vi "Finish.vi"   [LabVIEW 2018]
doc: "This VI is called just before exiting. It is expected to close I/O refnum, save collected data, etc."
uses:
  <vilib>/Rock Robotics/WPI/Utilities/WPI_GetSetVariantRefNum.vi
types:
  T1 = typedef "WPI_CompressorDevRef.ctl" = cluster{"DevStatus":errorcluster, "Pneumatics Control Module":u8}
  T2 = typedef "WPI_RobotDriveDevRef.ctl" = cluster{"DevStatus":errorcluster, "Motors[]":T3[], "Square Inputs":bool, "Max Output":dbl}
  T3 = typedef "WPI_MotorControlDeviceRef.ctl" = cluster{"DeviceStatus":errorcluster, "Type":T4, "PWM":cluster{"PWM Channel":T5, "DeadBand":T6}, "CAN":cluster{"Device Number":u8, "SetOutput VI Ref":variant, "GetOutput VI Ref":variant, "Enable VI Ref":variant, "Disable VI Ref":variant, "Data":variant}, "Invert":bool, "DIO PWM":cluster{"PWM \"Enable\" Channel":T5, "DIOChannel":T7, "PWM Rate":dbl}}
  T4 = typedef "WPI_MotorControlType.ctl" = enum16{"PWM", "CAN", "DIO PWM"}
  T5 = typedef "FPGA_DIOPWMChannel.ctl" = enum8{"PWM 0", "PWM 1", "PWM 2", "PWM 3", "PWM 4", "PWM 5", "PWM 6", "PWM 7", "PWM 8", "PWM 9", "PWM MXP 0", "PWM MXP 1", "PWM MXP 2", "PWM MXP 3", "PWM MXP 4", "PWM MXP 5", "PWM MXP 6", "PWM MXP 7", "PWM MXP 8", "PWM MXP 9", "Invalid"}
  T6 = typedef "WPI_PWMDeadband.ctl" = cluster{"Name":string, "maxPositivePwm":i32, "minPositivePwm":i32, "centerPwm":i32, "maxNegativePwm":i32, "minNegativePwm":i32, "angularRange":u16}
  T7 = typedef "FPGA_DIOChannel.ctl" = enum8{"DIO 0", "DIO 1", "DIO 2", "DIO 3", "DIO 4", "DIO 5", "DIO 6", "DIO 7", "DIO 8", "DIO 9", "DIO MXP 0", "DIO MXP 1", "DIO MXP 2", "DIO MXP 3", "DIO MXP 4", "DIO MXP 5", "DIO MXP 6", "DIO MXP 7", "DIO MXP 8", "DIO MXP 9", "DIO MXP 10", "DIO MXP 11", "DIO MXP 12", "DIO MXP 13", "DIO MXP 14", "DIO MXP 15", "SPI Port CS1", "SPI Port CS2", "SPI Port CS3", "SPI Port MISO", "SPI Port MOSI", "Invalid"}
  T8 = typedef "WPI_EncoderDevRef.ctl" = cluster{"DevStatus":errorcluster, "EncoderIndex":T9, "CounterIndex":T10, "DistancePerCount":dbl, "Decoding Type":T11}
  T9 = typedef "FPGA_EncoderIdx.ctl" = enum8{"Enc 0", "Enc 1", "Enc 2", "Enc 3", "Enc 4", "Enc 5", "Enc 6", "Enc 7", "Invalid"}
  T10 = typedef "FPGA_CounterCtrSystemIndex.ctl" = enum8{"Ctr 0", "Ctr 1", "Ctr 2", "Ctr 3", "Ctr 4", "Ctr 5", "Ctr 6", "Ctr 7", "Invalid"}
  T11 = typedef "WPI_EncoderType.ctl" = enum16{"1x", "2x", "4x"}
  T12 = typedef "WPI_SolenoidDevRef.ctl" = cluster{"DevStatus":errorcluster, "Pneumatics Control Module":u8, "Forward Solenoid Channel":T13, "Reverse Solenoid Channel":T13}
  T13 = typedef "WPI_SolenoidChannel.ctl" = enum8{"Solenoid 0", "Solenoid 1", "Solenoid 2", "Solenoid 3", "Solenoid 4", "Solenoid 5", "Solenoid 6", "Solenoid 7", "Invalid"}
  T14 = typedef "WPI_JoystickDevRef.ctl" = cluster{"Device":T15}
  T15 = typedef "WPI_JoystickDeviceEnum.ctl" = enum16{"USB 0", "USB 1", "USB 2", "USB 3", "USB 4", "USB 5"}
  T16 = typedef "WPI_DigitalInputDevRef.ctl" = cluster{"DevStatus":errorcluster, "DIO Channel":T7}
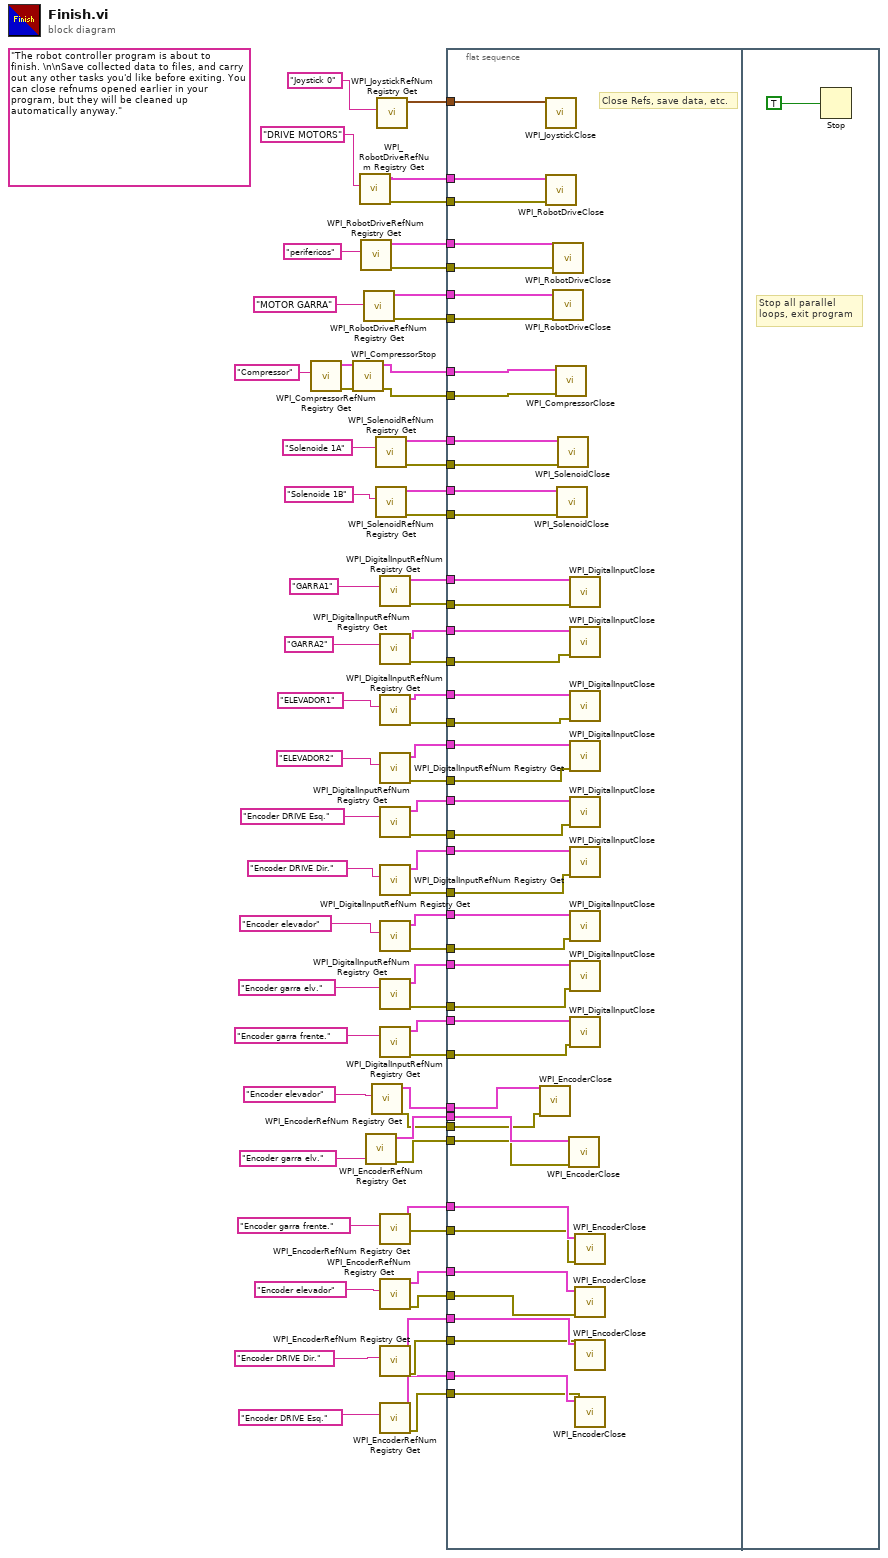
[diagram p0: block diagram]
diagram:
  (unwired) "The robot controller program is about to finish. \n\nSave collected data to files, and carry out any other tasks you'd like before exiting. You can close refnums opened earlier in your program, but they will be cleaned up automatically anyway."
  n1 = call <vilib>:"WPI_CompressorRefNum Registry Get.vi"("refnum name"="Compressor") -> ("error out"=w63:errorcluster, "CompressorDevRef"=w64:T1)  [unwired: 9 in]
  n2 = call <vilib>:"WPI_CompressorStop.vi"("error in (no error)"=w63, "CompressorDevRef"=w64) -> ("error out"=w61:errorcluster, "CompressorDevRef"=w60:T1)  [unwired: 8 in]
  n3 = call <vilib>:"WPI_RobotDriveRefNum Registry Get.vi"("refnum name"="DRIVE MOTORS") -> ("error out"=w4:errorcluster, "RobotDriveDevRef"=w11:T2)  [unwired: 9 in]
  n4 = call <vilib>:"WPI_RobotDriveRefNum Registry Get.vi"("refnum name"="perifericos") -> ("error out"=w3:errorcluster, "RobotDriveDevRef"=w8:T2)  [unwired: 9 in]
  n5 = call <vilib>:"WPI_RobotDriveRefNum Registry Get.vi"("refnum name"="MOTOR GARRA") -> ("error out"=w2:errorcluster, "RobotDriveDevRef"=w7:T2)  [unwired: 9 in]
  n6 = call <vilib>:"WPI_EncoderRefNum Registry Get.vi"("refnum name"="Encoder garra elv.") -> ("error out"=w33:errorcluster, "EncoderDevRef"=w34:T8)  [unwired: 9 in]
  n7 = call <vilib>:"WPI_EncoderRefNum Registry Get.vi"("refnum name"="Encoder elevador") -> ("error out"=w5:errorcluster, "EncoderDevRef"=w6:T8)  [unwired: 9 in]
  n8 = call <vilib>:"WPI_SolenoidRefNum Registry Get.vi"("refnum name"="Solenoide 1A") -> ("error out"=w58:errorcluster, "SolenoidDevRef"=w59:T12)  [unwired: 9 in]
  n9 = call <vilib>:"WPI_SolenoidRefNum Registry Get.vi"("refnum name"="Solenoide 1B") -> ("error out"=w55:errorcluster, "SolenoidDevRef"=w56:T12)  [unwired: 9 in]
  n10 = call <vilib>:"WPI_JoystickRefNum Registry Get.vi"("refnum name"="Joystick 0") -> ("JoystickDevRef"=w66:T14)  [unwired: 1 in, 9 out]
  n11 = call <vilib>:"WPI_DigitalInputRefNum Registry Get.vi"("refnum name"="GARRA1") -> ("error out"=w51:errorcluster, "DigitalInputDevRef"=w52:T16)  [unwired: 9 in]
  n12 = call <vilib>:"WPI_DigitalInputRefNum Registry Get.vi"("refnum name"="GARRA2") -> ("error out"=w49:errorcluster, "DigitalInputDevRef"=w50:T16)  [unwired: 9 in]
  n13 = call <vilib>:"WPI_DigitalInputRefNum Registry Get.vi"("refnum name"="ELEVADOR1") -> ("error out"=w47:errorcluster, "DigitalInputDevRef"=w48:T16)  [unwired: 9 in]
  n14 = call <vilib>:"WPI_DigitalInputRefNum Registry Get.vi"("refnum name"="ELEVADOR2") -> ("error out"=w45:errorcluster, "DigitalInputDevRef"=w46:T16)  [unwired: 9 in]
  n15 = call <vilib>:"WPI_DigitalInputRefNum Registry Get.vi"("refnum name"="Encoder DRIVE Esq.") -> ("error out"=w43:errorcluster, "DigitalInputDevRef"=w44:T16)  [unwired: 9 in]
  n16 = call <vilib>:"WPI_DigitalInputRefNum Registry Get.vi"("refnum name"="Encoder DRIVE Dir.") -> ("error out"=w41:errorcluster, "DigitalInputDevRef"=w42:T16)  [unwired: 9 in]
  n17 = call <vilib>:"WPI_DigitalInputRefNum Registry Get.vi"("refnum name"="Encoder elevador") -> ("error out"=w39:errorcluster, "DigitalInputDevRef"=w40:T16)  [unwired: 9 in]
  n18 = call <vilib>:"WPI_DigitalInputRefNum Registry Get.vi"("refnum name"="Encoder garra elv.") -> ("error out"=w37:errorcluster, "DigitalInputDevRef"=w38:T16)  [unwired: 9 in]
  n19 = call <vilib>:"WPI_DigitalInputRefNum Registry Get.vi"("refnum name"="Encoder garra frente.") -> ("error out"=w35:errorcluster, "DigitalInputDevRef"=w36:T16)  [unwired: 9 in]
  n20 = call <vilib>:"WPI_EncoderRefNum Registry Get.vi"("refnum name"="Encoder garra frente.") -> ("error out"=w31:errorcluster, "EncoderDevRef"=w32:T8)  [unwired: 9 in]
  n21 = call <vilib>:"WPI_EncoderRefNum Registry Get.vi"("refnum name"="Encoder elevador") -> ("error out"=w29:errorcluster, "EncoderDevRef"=w30:T8)  [unwired: 9 in]
  n22 = call <vilib>:"WPI_EncoderRefNum Registry Get.vi"("refnum name"="Encoder DRIVE Dir.") -> ("error out"=w27:errorcluster, "EncoderDevRef"=w28:T8)  [unwired: 9 in]
  n23 = call <vilib>:"WPI_EncoderRefNum Registry Get.vi"("refnum name"="Encoder DRIVE Esq.") -> ("error out"=w25:errorcluster, "EncoderDevRef"=w26:T8)  [unwired: 9 in]
  n24 = flat-sequence {
    tunnel: w11 -> [w110]
    tunnel: w66 -> [w109]
    tunnel: w61 -> [w108]
    tunnel: w60 -> [w107]
    tunnel: w59 -> [w106]
    tunnel: w58 -> [w105]
    tunnel: w56 -> [w104]
    tunnel: w55 -> [w103]
    tunnel: w52 -> [w102]
    tunnel: w51 -> [w101]
    tunnel: w50 -> [w100]
    tunnel: w49 -> [w99]
    tunnel: w48 -> [w98]
    tunnel: w47 -> [w97]
    tunnel: w46 -> [w96]
    tunnel: w45 -> [w95]
    tunnel: w44 -> [w94]
    tunnel: w43 -> [w93]
    tunnel: w42 -> [w92]
    tunnel: w41 -> [w91]
    tunnel: w40 -> [w90]
    tunnel: w39 -> [w89]
    tunnel: w38 -> [w88]
    tunnel: w37 -> [w87]
    tunnel: w36 -> [w86]
    tunnel: w35 -> [w85]
    tunnel: w34 -> [w84]
    tunnel: w33 -> [w83]
    tunnel: w32 -> [w82]
    tunnel: w31 -> [w81]
    tunnel: w30 -> [w80]
    tunnel: w29 -> [w79]
    tunnel: w28 -> [w78]
    tunnel: w27 -> [w77]
    tunnel: w26 -> [w76]
    tunnel: w25 -> [w75]
    tunnel: w8 -> [w74]
    tunnel: w7 -> [w73]
    tunnel: w6 -> [w72]
    tunnel: w5 -> [w71]
    tunnel: w4 -> [w70]
    tunnel: w3 -> [w69]
    tunnel: w2 -> [w68]
    frame #0 {
      # "Close Refs, save data, etc."
      n25 = call <vilib>:"WPI_EncoderClose.vi"("error in (no error)"=w71, "EncoderDevRef"=w72) -> ()  [unwired: 9 in, 1 out]
      n26 = call <vilib>:"WPI_JoystickClose.vi"("JoystickDevRef"=w109) -> ()  [unwired: 11 out]
      n27 = call <vilib>:"WPI_RobotDriveClose.vi"("error in (no error)"=w70, "RobotDriveDevRef"=w110) -> ()  [unwired: 10 out]
      n28 = call <vilib>:"WPI_RobotDriveClose.vi"("error in (no error)"=w69, "RobotDriveDevRef"=w74) -> ()  [unwired: 10 out]
      n29 = call <vilib>:"WPI_RobotDriveClose.vi"("error in (no error)"=w68, "RobotDriveDevRef"=w73) -> ()  [unwired: 10 out]
      n30 = call <vilib>:"WPI_CompressorClose.vi"("error in (no error)"=w108, "CompressorDevRef"=w107) -> ()  [unwired: 9 in, 1 out]
      n31 = call <vilib>:"WPI_SolenoidClose.vi"("error in (no error)"=w103, "SolenoidDevRef"=w104) -> ()  [unwired: 9 in, 1 out]
      n32 = call <vilib>:"WPI_SolenoidClose.vi"("error in (no error)"=w105, "SolenoidDevRef"=w106) -> ()  [unwired: 9 in, 1 out]
      n33 = call <vilib>:"WPI_EncoderClose.vi"("error in (no error)"=w83, "EncoderDevRef"=w84) -> ()  [unwired: 9 in, 1 out]
      n34 = call <vilib>:"WPI_DigitalInputClose.vi"("error in (no error)"=w101, "DigitalInputDevRef"=w102) -> ()  [unwired: 9 in, 1 out]
      n35 = call <vilib>:"WPI_DigitalInputClose.vi"("error in (no error)"=w99, "DigitalInputDevRef"=w100) -> ()  [unwired: 9 in, 1 out]
      n36 = call <vilib>:"WPI_DigitalInputClose.vi"("error in (no error)"=w97, "DigitalInputDevRef"=w98) -> ()  [unwired: 9 in, 1 out]
      n37 = call <vilib>:"WPI_DigitalInputClose.vi"("error in (no error)"=w95, "DigitalInputDevRef"=w96) -> ()  [unwired: 9 in, 1 out]
      n38 = call <vilib>:"WPI_DigitalInputClose.vi"("error in (no error)"=w93, "DigitalInputDevRef"=w94) -> ()  [unwired: 9 in, 1 out]
      n39 = call <vilib>:"WPI_DigitalInputClose.vi"("error in (no error)"=w91, "DigitalInputDevRef"=w92) -> ()  [unwired: 9 in, 1 out]
      n40 = call <vilib>:"WPI_DigitalInputClose.vi"("error in (no error)"=w89, "DigitalInputDevRef"=w90) -> ()  [unwired: 9 in, 1 out]
      n41 = call <vilib>:"WPI_DigitalInputClose.vi"("error in (no error)"=w87, "DigitalInputDevRef"=w88) -> ()  [unwired: 9 in, 1 out]
      n42 = call <vilib>:"WPI_DigitalInputClose.vi"("error in (no error)"=w85, "DigitalInputDevRef"=w86) -> ()  [unwired: 9 in, 1 out]
      n43 = call <vilib>:"WPI_EncoderClose.vi"("error in (no error)"=w81, "EncoderDevRef"=w82) -> ()  [unwired: 9 in, 1 out]
      n44 = call <vilib>:"WPI_EncoderClose.vi"("error in (no error)"=w79, "EncoderDevRef"=w80) -> ()  [unwired: 9 in, 1 out]
      n45 = call <vilib>:"WPI_EncoderClose.vi"("error in (no error)"=w77, "EncoderDevRef"=w78) -> ()  [unwired: 9 in, 1 out]
      n46 = call <vilib>:"WPI_EncoderClose.vi"("error in (no error)"=w75, "EncoderDevRef"=w76) -> ()  [unwired: 9 in, 1 out]
    }
    frame #1 {
      # "Stop all parallel\nloops, exit program"
      n47 = Stop(stop? (T)=TRUE ("Quit")) -> ()
    }
  }
